vi "wav converting test.vi"() -> ()   [LabVIEW 2020]
panel:
  out "x-y":dbl[](array[numeric])
  out "*(타입 *) &x 2":i32[](array[numeric]) format="%.0x"
  out "데이터 문자열":string
  out "32비트 정수":i32[](array[numeric]) format="%.0x"
  out "끼워넣기된 배열":u8[](array[numeric]) format="%.0x"
  out "*(타입 *) &x":fxp<+/-,24,24>[](array[numeric]) format="%.0x"
  out "x = y?":bool
  out "8비트 정수 2":i8[](array[numeric])
  out "8비트 정수":i8[](array[numeric])
  out "최소 인덱스":i32
  out "최소값":dbl format="%#.6f"
  out "최대 인덱스":i32
  out "최대값":dbl format="%#.6f"
  in  "offset":dbl format="%#_13g"
  in  "path":path caption="경로"
  in  "scale":dbl format="%#_13g"
  out "x*y":dbl[](array[numeric]) format="%#.6f"
  out "웨이브폼 그래프":dbl[][](graph)
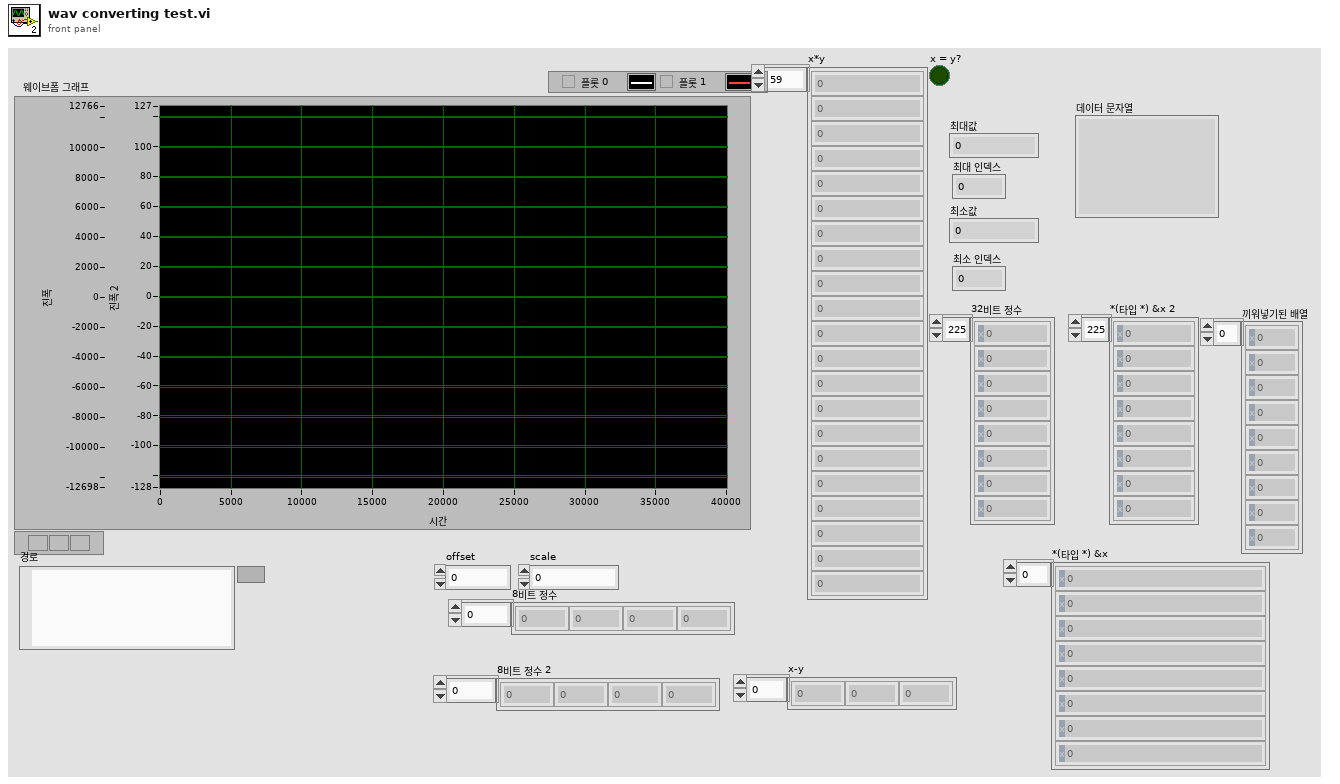
[diagram p1: front panel]
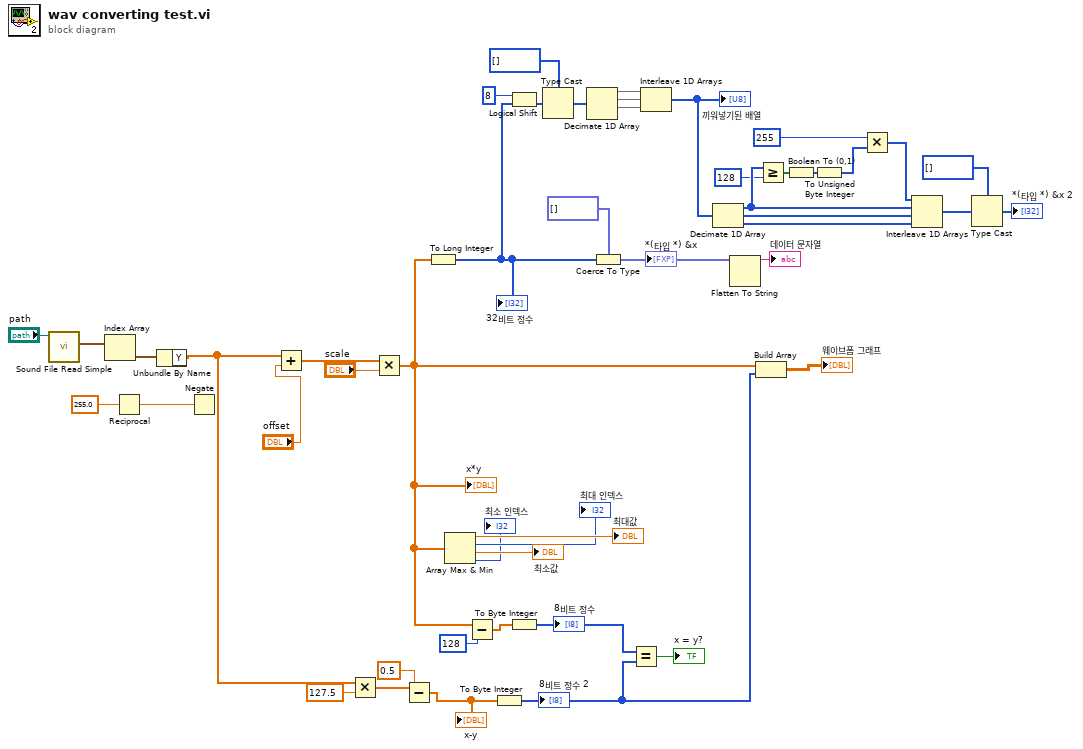
[diagram p0: block diagram]
diagram:
  n1 = call <vilib>:"Sound File Read Simple.vi"("path"="path") -> ("data"=w46:waveform(dbl)[])  [unwired: 7 in, 3 out]
  n2 = Index Array(array=w46) -> (element=w45:waveform(dbl))  [unwired: 1 in]
  n3 = Reciprocal(x=255.0) -> (1/x=w2:dbl)
  n4 = Unbundle By Name(w45) -> ("Y"=w5:dbl[])
  n5 = Negate(x=w2) -> ()  [unwired: 1 out]
  n6 = Add(x=w5, y="offset") -> (x+y=w47:dbl[])
  n7 = Multiply(x=w5, y=127.5) -> (x*y=w36:dbl[])
  n8 = Multiply(x=w47, y="scale") -> (x*y=w6:dbl[])
  "x*y" <- w6
  n9 = Subtract(x=w36, y=0.5) -> (x-y=w34:dbl[])
  "x-y" <- w34
  n10 = To Long Integer(number=w6) -> (32bit integer=w28:i32[])
  "32비트 정수" <- w28
  n11 = Array Max & Min(array=w6) -> (max value=→"최대값":dbl, max index (indices)=→"최대 인덱스":i32, min value=→"최소값":dbl, min index (indices)=→"최소 인덱스":i32)
  n12 = Subtract(x=w6, y=u8 128) -> (x-y=w39:dbl[])
  n13 = To Byte Integer(number=w34) -> (8bit integer=w4:i8[])
  "8비트 정수 2" <- w4
  n14 = Logical Shift(y=i16 8, x=w28) -> (x << y=w25:i32[])
  n15 = To Byte Integer(number=w39) -> (8bit integer=w33:i8[])
  "8비트 정수" <- w33
  n16 = Type Cast(type=u8[] [], x=w25) -> (*(type *) &x=w26:u8[])
  n17 = Decimate 1D Array(w26) -> (w23:u8[], w22:u8[], w21:u8[])  [unwired: 1 out]
  n18 = Coerce To Type(0:w28, 1:fxp<+/-,24,24>[] []) -> (2:w30:fxp<+/-,24,24>[])
  "*(타입 *) &x" <- w30
  n19 = Equal?(x=w33, y=w4) -> (x = y?=→"x = y?":bool)
  n20 = Interleave 1D Arrays(w23, w22, w21) -> (w20:u8[])
  "끼워넣기된 배열" <- w20
  n21 = Decimate 1D Array(w20) -> (w17:u8[], w19:u8[], w18:u8[])
  n22 = Flatten To String(anything=w30) -> (data string=→"데이터 문자열":string)  [unwired: 3 in, 2 out]
  n23 = Build Array(w6, w4) -> (→"웨이브폼 그래프":dbl[][])
  n24 = Greater Or Equal?(x=w17, y=u8 128) -> (x >= y?=w14:bool[])
  n25 = Boolean To (0,1)(Boolean=w14) -> (0, 1=w13:i16[])
  n26 = To Unsigned Byte Integer(number=w13) -> (unsigned 8bit integer=w12:u8[])
  n27 = Multiply(x=u8 255, y=w12) -> (x*y=w11:u8[])
  n28 = Interleave 1D Arrays(w11, w17, w19, w18) -> (w10:u8[])
  n29 = Type Cast(type=i32[] [], x=w10) -> (*(type *) &x=→"*(타입 *) &x 2":i32[])
